vi "Get_Timestamp.vi"() -> (0 "Timestamp":string)   [LabVIEW 2011]
doc: "This VI generates a timestamp using the current date and time that is suitable for use in a file name."
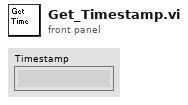
[diagram p1: front panel]
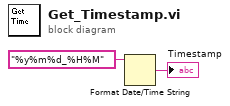
[diagram p0: block diagram]
diagram:
  n1 = Format Date/Time String(time format string (%c)="%y%m%d_%H%M") -> (date/time string=→"Timestamp":string)  [unwired: 2 in]
